vi "macro_DoubleSolenoid_Pulse_Execute.vi"() -> ()   [LabVIEW 2019, in "Trajectory_Library.lvlib"]
uses:
  Trajectory_Library.lvlib
  <vilib>/Rock Robotics/WPI/Solenoid/WPI_SolenoidValue.ctl
panel:
  out "Solenoid Cmd":T1
  in  "Robot Enabled":bool
  in  "Solenoid Demand":bool
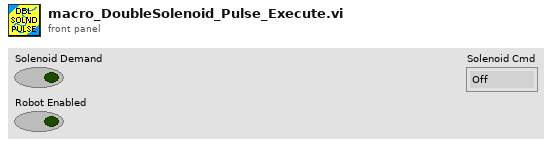
[diagram p1: front panel]
types:
  T1 = typedef "WPI_SolenoidValue.ctl" = enum16{"Off", "On", "Forward", "Reverse"}
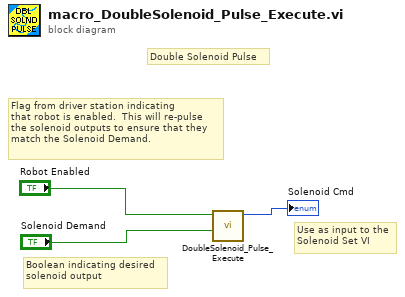
[diagram p0: block diagram]
diagram:
  # "Flag from driver station indicating\nthat robot is enabled.  This will re-pulse\nthe solenoid outputs to ensure that they\nmatch the Solenoid Demand."
  # "Boolean indicating desired\nsolenoid output"
  # "Use as input to the\nSolenoid Set VI"
  # "Double Solenoid Pulse"
  n1 = call "DoubleSolenoid_Pulse_Execute.vi"("Solenoid Demand"="Solenoid Demand", "Robot Enabled"="Robot Enabled") -> ("Solenoid Cmd"=→"Solenoid Cmd":T1)  [unwired: 9 in]
